vi "预处理部分.vi"(0 "mono 16-bit":dbl[][](array[numeric])) -> (1 "y":dbl[][](array[numeric]), 2 "s1":dbl, 3 "s2":dbl, 4 "波形图 2":dbl[][](graph))   [LabVIEW 2018]
panel:
  out "波形图":dbl[][](graph)
  out "error out":errorcluster
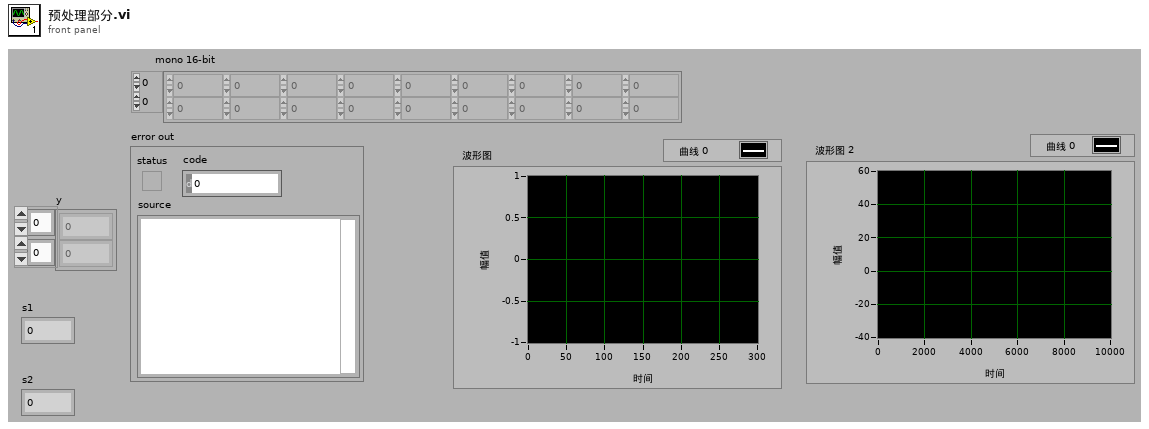
[diagram p1: front panel]
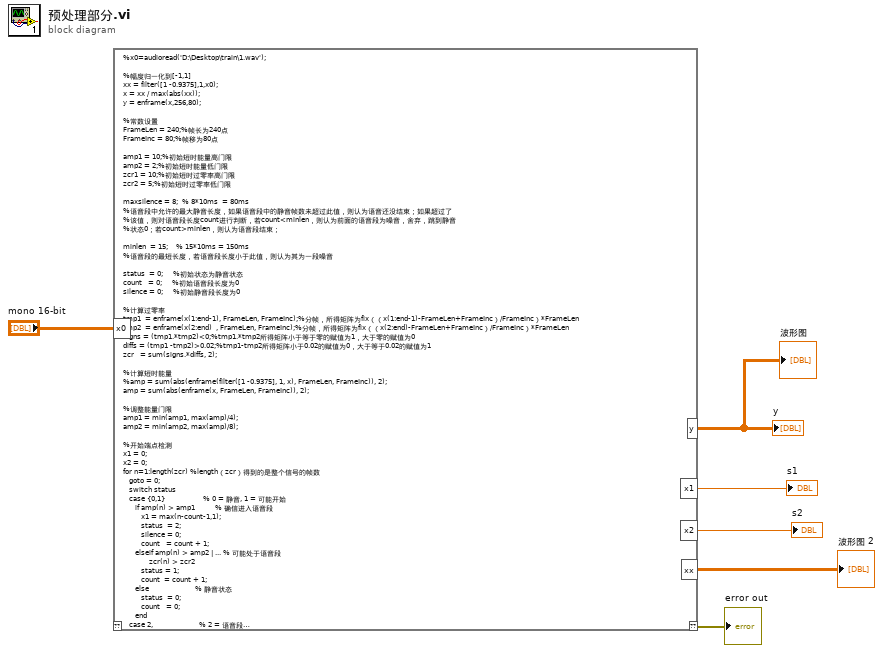
[diagram p0: block diagram]
diagram:
  n1 = script code="%x0=audioread('D:\\Desktop\\train\\1.wav');\n\n%幅度归一化到[-1,1]\nxx = filter([1 -0.9375],1,x0);\nx = xx / max(abs(xx));\ny = enframe(x,256,80);\n\n%常数设置\nFrameLen = 240;%帧长为240点\nFrameInc = 80;%帧移为80点\n \namp1 = 10;%初始短时能量高门限\namp2 = 2;%初始短时能量低门限\nzcr1 = 10;%初始短时过零率高门限\nzcr2 = 5;%初始短时过零率低门限\n \nmaxsilence = 8;  % 8*10ms  = 80ms\n%语音段中允许的最大静音长度，如果语音段中的静音帧数未超过此值，则认为语音还没结束；如果超过了\n%该值，则对语音段长度count进行判断，若count<minlen，则认为前面的语音段为噪音，舍弃，跳到静音\n%状态0；若count>minlen，则认为语音段结束；\n\nminlen  = 15;    % 15*10ms = 150ms\n%语音段的最短长度，若语音段长度小于此值，则认为其为一段噪音\n\nstatus  = 0;     %初始状态为静音状态\ncount   = 0;     %初始语音段长度为0\nsilence = 0;     %初始静音段长度为0\n \n%计算过零率\ntmp1  = enframe(x(1:end-1), FrameLen, FrameInc);%分帧，所得矩阵为fix（（x(1:end-1)-FrameLen+FrameInc）/FrameInc）*FrameLen\ntmp2  = enframe(x(2:end)  , FrameLen, FrameInc);%分帧，所得矩阵为fix（（x(2:end)-FrameLen+FrameInc）/FrameInc）*FrameLen\nsigns = (tmp1.*tmp2)<0;%tmp1.*tmp2所得矩阵小于等于零的赋值为1，大于零的赋值为0\ndiffs = (tmp1 -tmp2)>0.02;%tmp1-tmp2所得矩阵小于0.02的赋值为0，大于等于0.02的赋值为1\nzcr   = sum(signs.*diffs, 2);\n \n%计算短时能量\n%amp = sum(abs(enframe(filter([1 -0.9375], 1, x), FrameLen, FrameInc)), 2);\namp = sum(abs(enframe(x, FrameLen, FrameInc)), 2);\n \n%调整能量门限\namp1 = min(amp1, max(amp)/4);\namp2 = min(amp2, max(amp)/8);\n \n%开始端点检测\nx1 = 0;\nx2 = 0;\nfor n=1:length(zcr) %length（zcr）得到的是整个信号的帧数\n   goto = 0;\n   switch status\n   case {0,1}                   % 0 = 静音, 1 = 可能开始\n      if amp(n) > amp1          % 确信进入语音段\n         x1 = max(n-count-1,1);\n         status  = 2;\n         silence = 0;\n         count   = count + 1;\n      elseif amp(n) > amp2 | ... % 可能处于语音段\n             zcr(n) > zcr2\n         status = 1;\n         count  = count + 1;\n      else                       % 静音状态\n         status  = 0;\n         count   = 0;\n      end\n   case 2,                       % 2 = 语音段\n      if amp(n) > amp2 | ...     % 保持在语音段\n         zcr(n) > zcr2\n         count = count + 1;\n      else                       % 语音将结束\n         silence = silence+1;\n         if silence < maxsilence % 静音还不够长，尚未结束\n            count  = count + 1;\n         elseif count < minlen   % 语音长度太短，认为是噪声\n            status  = 0;\n            silence = 0;\n            count   = 0;\n         else                    % 语音结束\n            status  = 3;\n         end\n      end\n   case 3,\n      break;\n   end\nend  \ncount = count-silence/2;\nx2 = x1 + count -1;\n%xx2 = x((x1-1)*80+1:(x2-1)*80+256);"("x0"="mono 16-bit") -> ("??"=→"error out":errorcluster, "y"=→"y" →"波形图":dbl[][], "x1"=→"s1":dbl, "x2"=→"s2":dbl, "xx"=→"波形图 2":dbl[][])  [unwired: 1 in]
